vi "MSScript_Calc_ArrayInit.vi"(6 "Value Error?":bool[](array[boolean]), 8 "ArrayVariable in":ext[](array[numeric]), 9 "Param Items":i32) -> (0 "ArrayVariable out":ext[](array[numeric]), 2 "CmdError?":bool)   [LabVIEW 2018, in "MSScript.lvclass"]
uses:
  MSScript.lvclass
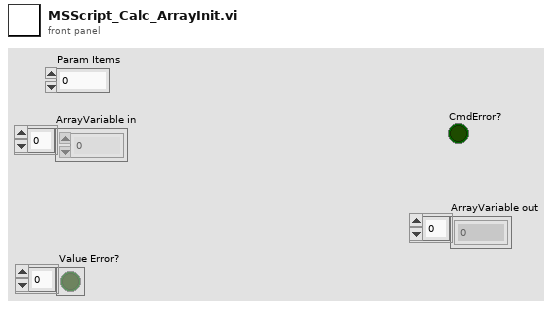
[diagram p1: front panel]
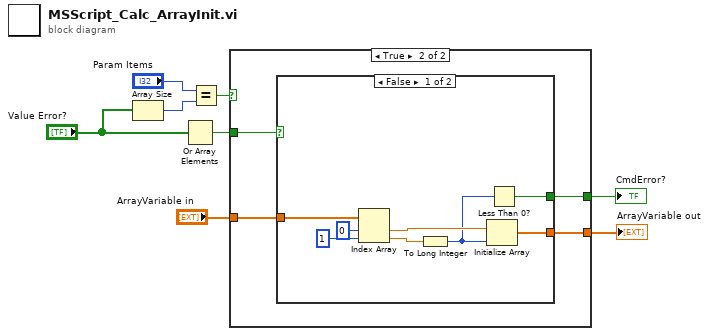
[diagram p0: block diagram]
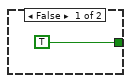
[diagram p2: hidden frame]
diagram:
  n1 = Array Size(array="Value Error?") -> (size(s)=w5:i32)
  n2 = Or Array Elements(Boolean array="Value Error?") -> (logical OR=w7:bool)
  n3 = Equal?(x="Param Items", y=w5) -> (x = y?=w3:bool)
  n4 = case shown="True" w3 {
    tunnel: [TRUE w10] -> w2
    tunnel: w7 -> [_ w13]
    tunnel: [_ w11] -> w8
    tunnel: "ArrayVariable in" -> [_ w12]
    frame False {
    }
    frame True {
      n5 = case shown="False" w13 {
        tunnel: w12 -> [w21 _]
        tunnel: [w16 _] -> w11
        tunnel: [w14 _] -> w10
        frame False {
          n6 = Index Array(array=w21, index #1=0 ("index"), index #2=1 ("index")) -> (element #1=w18:ext, element #2=w17:ext)
          n7 = To Long Integer(number=w17) -> (32bit integer=w15:i32)
          n8 = Initialize Array(w18, w15) -> (w16:ext[])
          n9 = Less Than 0?(x=w15) -> (x < 0?=w14:bool)
        }
        frame True {
        }
      }
    }
  }
  "ArrayVariable out" <- w8
  "CmdError?" <- w2
